vi "Calibration Dialog.vi"(8 "error in (no error)":errorcluster) -> (0 "error out":errorcluster, 2 "Cancelled?":bool, 3 "Cal Select":string)   [LabVIEW 2024]
doc: "Dialog for selecting user specified settings."
panel:
  in  "Calibration Select":enum16{"Bridge Offset Nulling"}(ring)
  in  "Cancel Button":bool
  in  "OK Button":bool
  # "Non visible portion of dialog (needed for connector pane)."
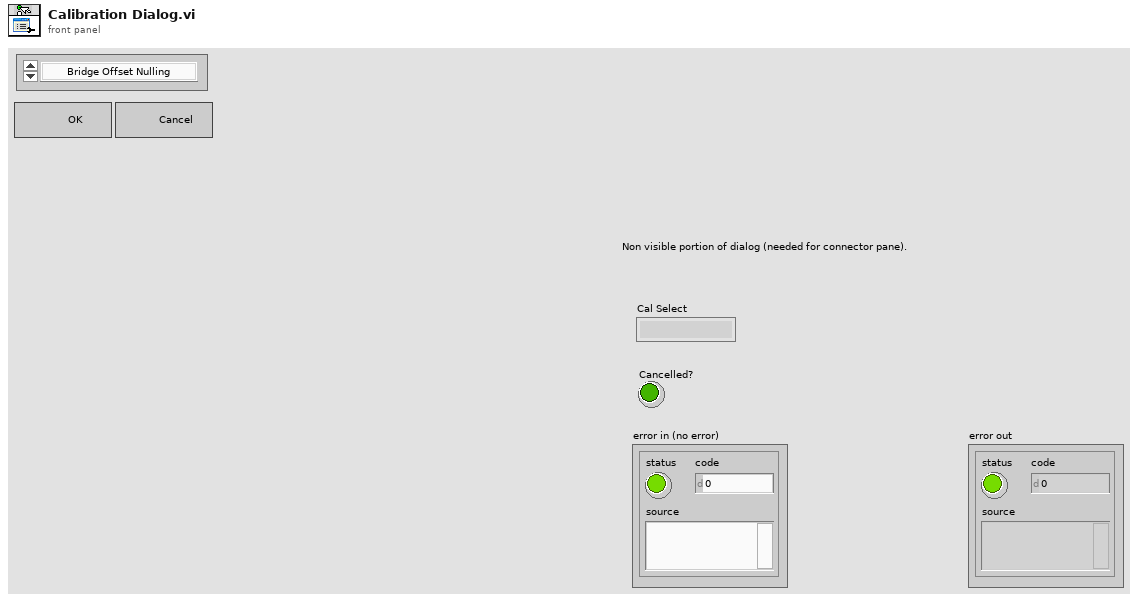
[diagram p1: front panel]
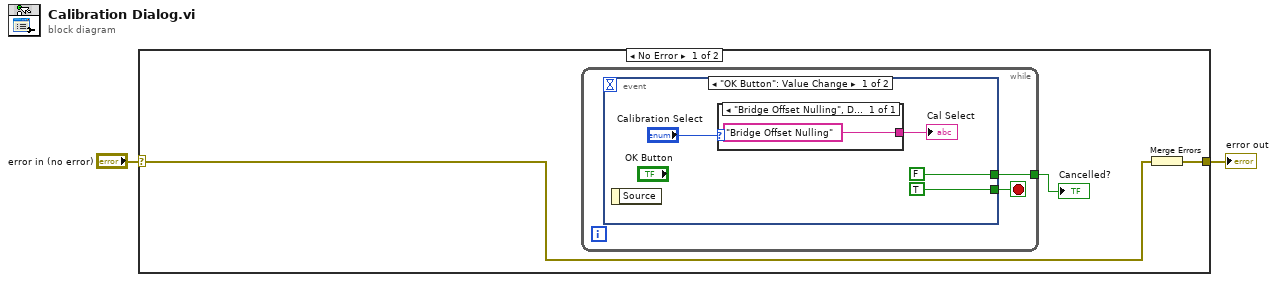
[diagram p0: block diagram]
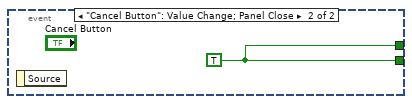
[diagram p2: hidden frame]
diagram:
  n1 = case shown="No Error" "error in (no error)" {
    selector: "error in (no error)" -> [w3 w14]
    tunnel: [w4 w14] -> w2
    frame No Error {
      n2 = while {
        tunnel: [w6] -> w5
        stop <- w7 stop-if-true
        n3 = event shown="[0] \"OK Button\": Value Change" {
          selector: _ -> [_ _]
          dyn-events: _ -> [_ _]
          timeout: _ -> [_ _]
          tunnel: [TRUE w13] -> w7
          tunnel: [FALSE w13] -> w6
          event "OK Button": Value Change {
            n4 = event-data() -> ()  [unwired: 1 in, 1 out]
            n5 = case shown="\"Bridge Offset Nulling\", Default" "Calibration Select" {
              tunnel: ["Bridge Offset Nulling"] -> w8
              frame "Bridge Offset Nulling", Default {
              }
            }
            "Cal Select" <- w8
          }
          event "Cancel Button": Value Change; Panel Close {
            w13 = TRUE
            n6 = event-data() -> ()  [unwired: 1 in, 1 out]
          }
        }
      }
      "Cancelled?" <- w5
      n7 = Merge Errors(w3) -> (w4:errorcluster)
    }
    frame Error {
    }
  }
  "error out" <- w2
